vi "ThermoCouple_DAQ.vi"(6 "Temps in":dbl[](array[numeric]), 7 "Setup":T1, 8 "error in (no error)":errorcluster, 9 "Data in":cluster{"Temps":dbl[][], "Gradients":dbl[][]}, 10 "Period (ms)":i64, 11 "samples":i32) -> (0 "error out":errorcluster, 1 "Gradients graph":waveform(dbl)[](array[waveform]), 2 "Temps out":dbl[](array[numeric]), 3 "Data out":cluster{"Temps":dbl[][], "Gradients":dbl[][]}, 4 "stop?":bool, 5 "Temps graph":waveform(dbl)[](array[waveform]))   [LabVIEW 2022 SP3]
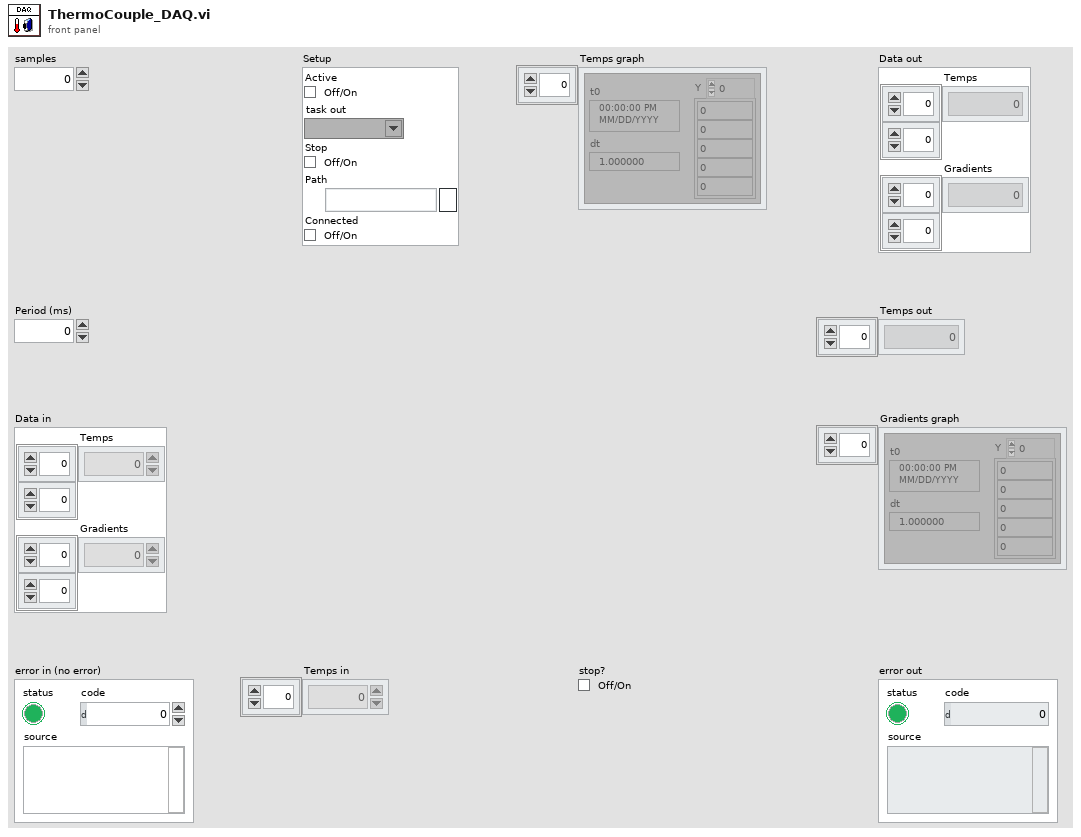
[diagram p1: front panel]
types:
  T1 = cluster{"Active":bool, "task out":refnum<k21>, "Stop":bool, "Path":path, "Connected":bool}
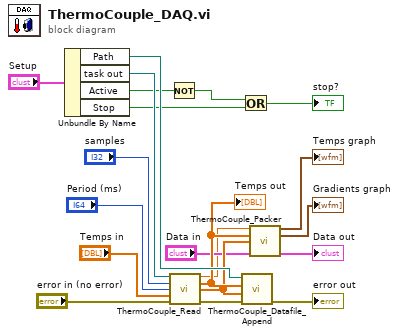
[diagram p0: block diagram]
diagram:
  n1 = Unbundle By Name("Setup") -> ("Path"=w20:path, "task out"=w13:refnum<k21>, "Active"=w4:bool, "Stop"=w2:bool)
  n2 = Not(x=w4) -> (.not. x?=w5:bool)
  n3 = call "ThermoCouple_Read.vi"("task"=w13, "samples"="samples", "period (ms)"="Period (ms)", "prev Temps"="Temps in", "error in"="error in (no error)") -> ("dt"=w8:dbl, "Temps"=w19:dbl[], "Gradients"=w18:dbl[], "error out"=w16:errorcluster)  [unwired: 7 in]
  "Temps out" <- w19
  n4 = Or(x=w5, y=w2) -> (x .or. y?=→"stop?":bool)
  n5 = call "ThermoCouple_Datafile_Append.vi"("error in"=w16, "Gradients"=w18, "Temps"=w19, "Path"=w20) -> ("error out"=→"error out":errorcluster)  [unwired: 7 in]
  n6 = call "ThermoCouple_Packer.vi"("dt"=w8, "Temps in"=w19, "Gradients in"=w18, "Data in"="Data in") -> ("Temps"=→"Temps graph":waveform(dbl)[], "Gradients"=→"Gradients graph":waveform(dbl)[], "Data out"=→"Data out":cluster{"Temps":dbl[][], "Gradients":dbl[][]})  [unwired: 9 in]
